vi "slm_control_MAIN.vi"() -> ()   [LabVIEW 2024]
uses:
  <vilib>/Python/Open Anaconda Python Session.vi
panel:
  in  "Send to SLM":bool=TRUE
  in  "stop_all":bool
  in  "Laser Wavelength":i32=635
  in  "SLM Cols":i32=800
  in  "SLM Rows":i32=600
  out "SLM Display":T1(plugin-control)
  in  "Tab Control":enum32{"Double Pass", "Single Pass"}(tab)
  in  "Linear Period Y":dbl
  in  "Linear Period X":dbl=4.0
  in  "Y Offset B":i32 min=-150 max=150 step=1
  in  "Y Offset A":i32 min=-150 max=150 step=1
  in  "X Offset A":i32 min=-150 max=150 step=1
  in  "B Display":bool=TRUE
  in  "A Display":bool=TRUE
  in  "Modulation Mode Double Pass":string(combo)
  in  "X Offset B":i32 min=-150 max=150 step=1
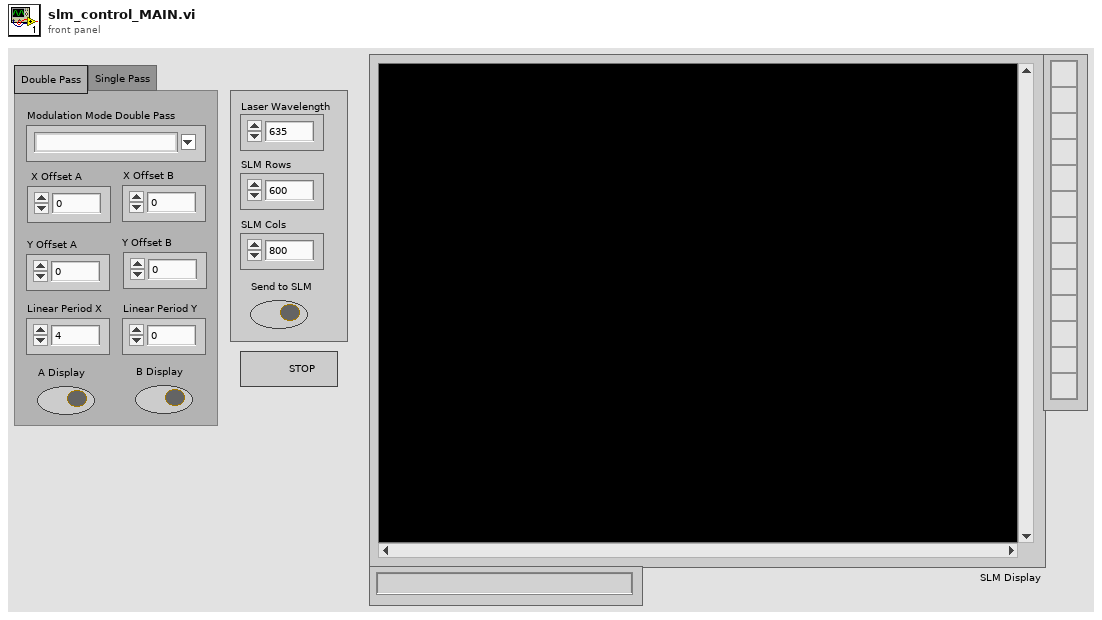
[diagram p1: front panel]
types:
  T1 = typedef "IMAQ Image.ctl" = refnum<image>
  T2 = enum16{"Init", "Idle", "Compute Modulation", "Stop All", "Shift Modulation"}
  T3 = enum16{"Init", "Idle", "Compute Modulation", "Stop All"}
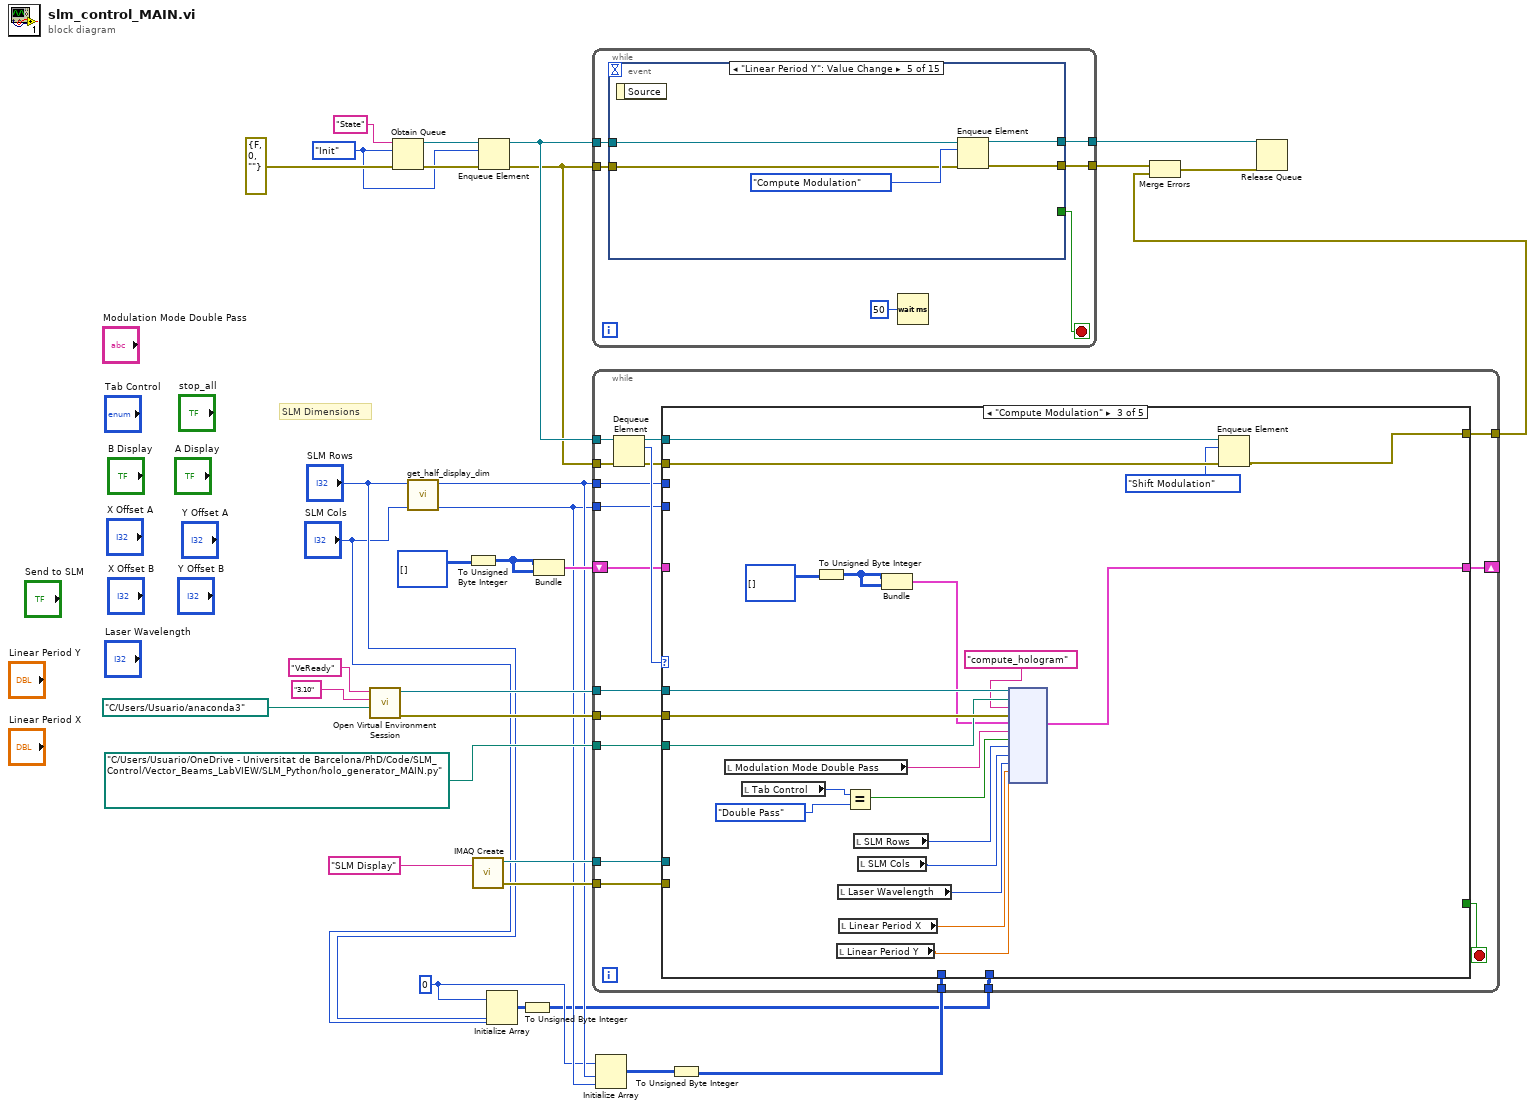
[diagram p0: block diagram]
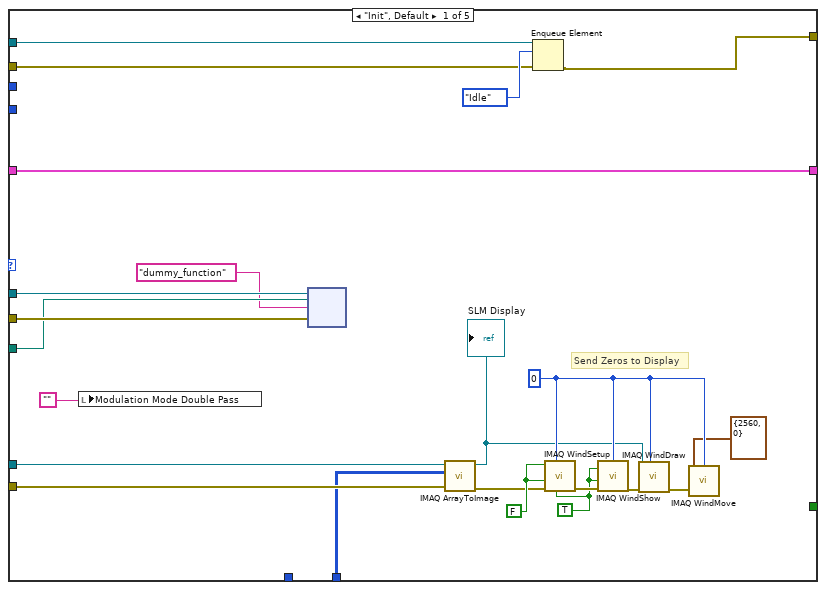
[diagram p2: hidden frame]
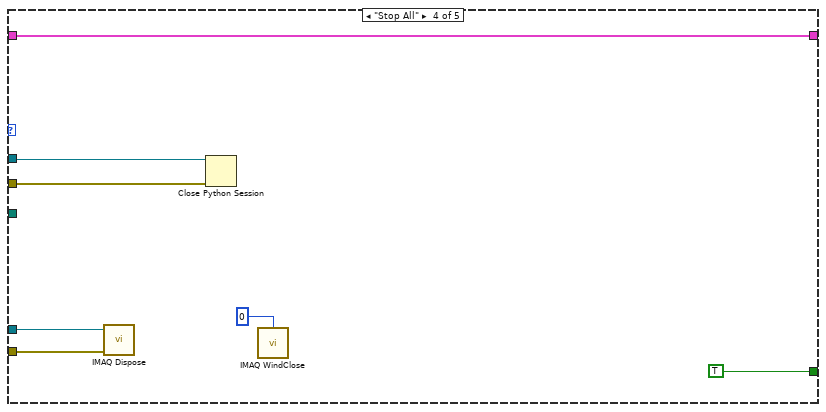
[diagram p4: hidden frame]
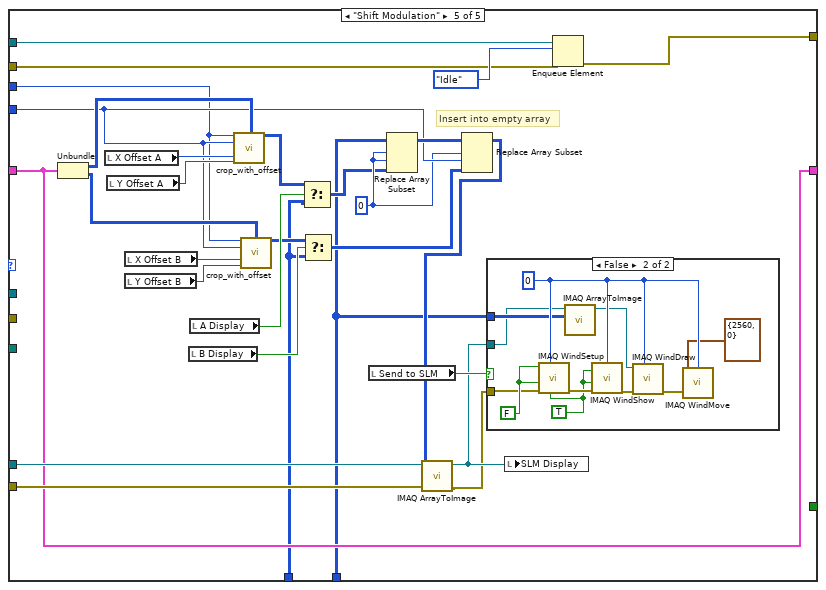
[diagram p5: hidden frame]
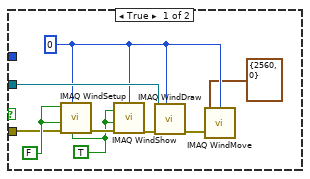
[diagram p6: hidden frame]
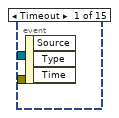
[diagram p7: hidden frame]
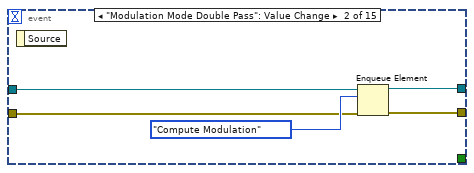
[diagram p8: hidden frame]
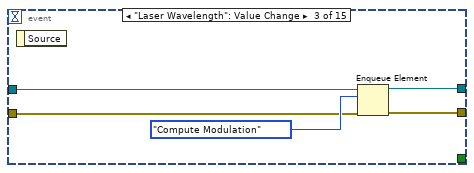
[diagram p9: hidden frame]
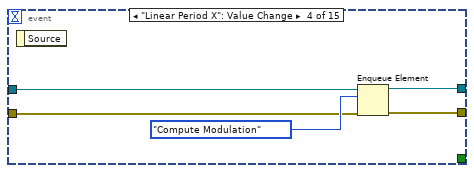
[diagram p10: hidden frame]
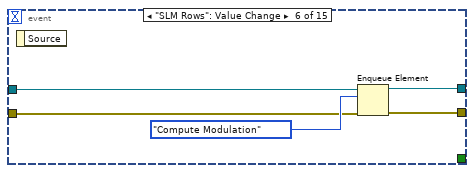
[diagram p11: hidden frame]
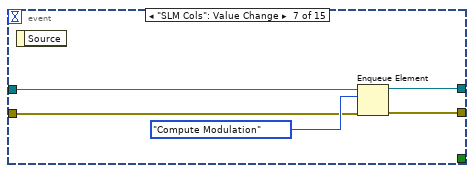
[diagram p12: hidden frame]
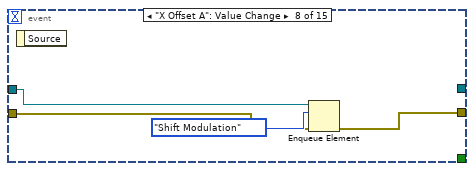
[diagram p13: hidden frame]
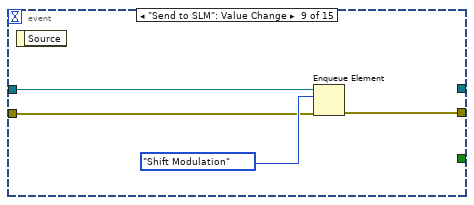
[diagram p14: hidden frame]
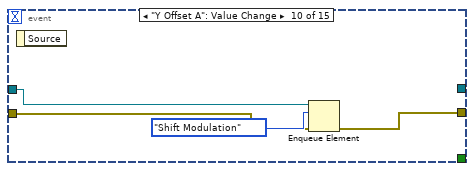
[diagram p15: hidden frame]
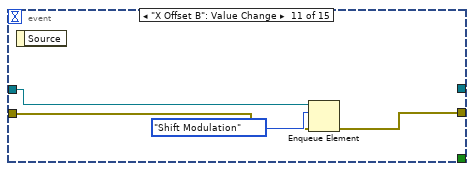
[diagram p16: hidden frame]
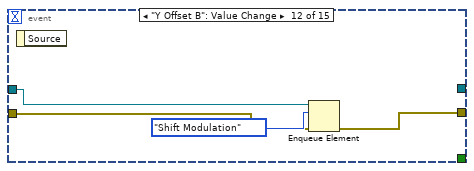
[diagram p17: hidden frame]
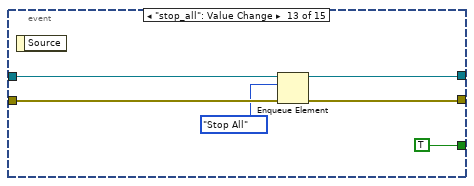
[diagram p18: hidden frame]
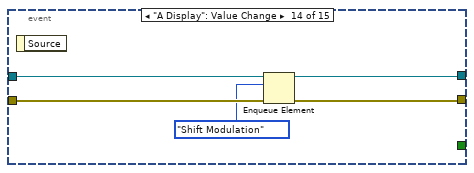
[diagram p19: hidden frame]
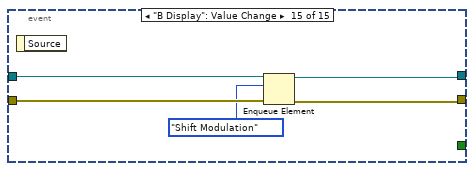
[diagram p20: hidden frame]
diagram:
  w5 = 0
  w9 = T2."Init"
  # "SLM Dimensions"
  n1 = call-poly <vilib>:"Open Virtual Environment Session.vi"("Anaconda path"=path "C:/Users/Usuario/anaconda3", "Python version"="3.10", "Env name"="VeReady") -> ("error out"=w23:errorcluster, "session out"=w24:refnum<k35>)  [unwired: 7 in]
  n2 = Obtain Queue(name (unnamed)="State", element data type=w9, error in (no error)=errorcluster {"status"=FALSE, "code"=0, "source"=""}) -> (queue out=w13:refnum<queue>, error out=w11:errorcluster)  [unwired: 2 in, 1 out]
  n3 = call "get_half_display_dim.vi"("Cols"="SLM Cols", "Rows"="SLM Rows") -> ("Semi Cols"=w6:i32, "Semi Rows"=w7:i32)  [unwired: 8 in]
  n4 = To Unsigned Byte Integer(number=i32[][] []) -> (unsigned 8bit integer=w16:u8[][])
  n5 = call "IMAQ Create"("Image Name"="SLM Display") -> ("New Image"=w19:T1, "error out"=w18:errorcluster)  [unwired: 4 in]
  n6 = Enqueue Element(queue=w13, element=w9, error in (no error)=w11) -> (queue out=w12:refnum<queue>, error out=w10:errorcluster)  [unwired: 1 in, 1 out]
  n7 = Initialize Array(w5, "SLM Rows", "SLM Cols") -> (w14:i32[][])
  n8 = To Unsigned Byte Integer(number=w14) -> (unsigned 8bit integer=w1:u8[][])
  n9 = Bundle(w16, w16) -> (w15:cluster{u8[][], u8[][]})  [unwired: 1 in]
  n10 = while {
    tunnel: w12 -> [w36]
    tunnel: [w35] -> w31
    tunnel: [w34] -> w29
    tunnel: w10 -> [w33]
    stop <- w37 stop-if-true
    n11 = event shown="[4] \"Linear Period Y\": Value Change" {
      selector: _ -> [_ _ _ _ _ _ _ _ _ _ _ _ _ _ _]
      dyn-events: _ -> [_ _ _ _ _ _ _ _ _ _ _ _ _ _ _]
      timeout: _ -> [_ _ _ _ _ _ _ _ _ _ _ _ _ _ _]
      tunnel: [_ _ _ _ _ _ _ _ _ _ _ _ TRUE _ _] -> w37
      tunnel: w36 -> [_ w43 w48 w53 w58 w63 w68 w71 w75 w79 w83 w87 w93 w99 w104]
      tunnel: [_ w42 w47 w52 w57 w62 w67 _ _ _ _ _ w90 w98 w103] -> w35
      tunnel: [_ w41 w46 w51 w56 w61 w66 w69 w73 w77 w81 w85 w91 w96 w101] -> w34
      tunnel: w33 -> [_ w39 w44 w49 w54 w59 w64 w70 w74 w78 w82 w86 w92 w97 w102]
      event Timeout {
        n12 = event-data() -> ()  [unwired: 1 in, 3 out]
      }
      event "Modulation Mode Double Pass": Value Change {
        n13 = event-data() -> ()  [unwired: 1 in, 1 out]
        n14 = Enqueue Element(queue=w43, element=enum16{"Init", "Idle", "Compute Modulation"}."Compute Modulation", error in (no error)=w39) -> (queue out=w42:refnum<queue>, error out=w41:errorcluster)  [unwired: 1 in, 1 out]
      }
      event "Laser Wavelength": Value Change {
        n15 = event-data() -> ()  [unwired: 1 in, 1 out]
        n16 = Enqueue Element(queue=w48, element=enum16{"Init", "Idle", "Compute Modulation"}."Compute Modulation", error in (no error)=w44) -> (queue out=w47:refnum<queue>, error out=w46:errorcluster)  [unwired: 1 in, 1 out]
      }
      event "Linear Period X": Value Change {
        n17 = event-data() -> ()  [unwired: 1 in, 1 out]
        n18 = Enqueue Element(queue=w53, element=enum16{"Init", "Idle", "Compute Modulation"}."Compute Modulation", error in (no error)=w49) -> (queue out=w52:refnum<queue>, error out=w51:errorcluster)  [unwired: 1 in, 1 out]
      }
      event "Linear Period Y": Value Change {
        n19 = event-data() -> ()  [unwired: 1 in, 1 out]
        n20 = Enqueue Element(queue=w58, element=enum16{"Init", "Idle", "Compute Modulation"}."Compute Modulation", error in (no error)=w54) -> (queue out=w57:refnum<queue>, error out=w56:errorcluster)  [unwired: 1 in, 1 out]
      }
      event "SLM Rows": Value Change {
        n21 = event-data() -> ()  [unwired: 1 in, 1 out]
        n22 = Enqueue Element(queue=w63, element=enum16{"Init", "Idle", "Compute Modulation"}."Compute Modulation", error in (no error)=w59) -> (queue out=w62:refnum<queue>, error out=w61:errorcluster)  [unwired: 1 in, 1 out]
      }
      event "SLM Cols": Value Change {
        n23 = event-data() -> ()  [unwired: 1 in, 1 out]
        n24 = Enqueue Element(queue=w68, element=enum16{"Init", "Idle", "Compute Modulation"}."Compute Modulation", error in (no error)=w64) -> (queue out=w67:refnum<queue>, error out=w66:errorcluster)  [unwired: 1 in, 1 out]
      }
      event "X Offset A": Value Change {
        n25 = event-data() -> ()  [unwired: 1 in, 1 out]
        n26 = Enqueue Element(queue=w71, element=T2."Shift Modulation", error in (no error)=w70) -> (error out=w69:errorcluster)  [unwired: 1 in, 2 out]
      }
      event "Send to SLM": Value Change {
        n27 = event-data() -> ()  [unwired: 1 in, 1 out]
        n28 = Enqueue Element(queue=w75, element=T2."Shift Modulation", error in (no error)=w74) -> (error out=w73:errorcluster)  [unwired: 1 in, 2 out]
      }
      event "Y Offset A": Value Change {
        n29 = event-data() -> ()  [unwired: 1 in, 1 out]
        n30 = Enqueue Element(queue=w79, element=T2."Shift Modulation", error in (no error)=w78) -> (error out=w77:errorcluster)  [unwired: 1 in, 2 out]
      }
      event "X Offset B": Value Change {
        n31 = event-data() -> ()  [unwired: 1 in, 1 out]
        n32 = Enqueue Element(queue=w83, element=T2."Shift Modulation", error in (no error)=w82) -> (error out=w81:errorcluster)  [unwired: 1 in, 2 out]
      }
      event "Y Offset B": Value Change {
        n33 = event-data() -> ()  [unwired: 1 in, 1 out]
        n34 = Enqueue Element(queue=w87, element=T2."Shift Modulation", error in (no error)=w86) -> (error out=w85:errorcluster)  [unwired: 1 in, 2 out]
      }
      event "stop_all": Value Change {
        n35 = event-data() -> ()  [unwired: 1 in, 1 out]
        n36 = Enqueue Element(queue=w93, element=T3."Stop All", error in (no error)=w92) -> (queue out=w90:refnum<queue>, error out=w91:errorcluster)  [unwired: 1 in, 1 out]
      }
      event "A Display": Value Change {
        n37 = event-data() -> ()  [unwired: 1 in, 1 out]
        n38 = Enqueue Element(queue=w99, element=T2."Shift Modulation", error in (no error)=w97) -> (queue out=w98:refnum<queue>, error out=w96:errorcluster)  [unwired: 1 in, 1 out]
      }
      event "B Display": Value Change {
        n39 = event-data() -> ()  [unwired: 1 in, 1 out]
        n40 = Enqueue Element(queue=w104, element=T2."Shift Modulation", error in (no error)=w102) -> (queue out=w103:refnum<queue>, error out=w101:errorcluster)  [unwired: 1 in, 1 out]
      }
    }
    n41 = Wait (ms)(milliseconds to wait=u32 50) -> ()  [unwired: 1 out]
  }
  n42 = Initialize Array(w5, w7, w6) -> (w8:i32[][])
  n43 = To Unsigned Byte Integer(number=w8) -> (unsigned 8bit integer=w4:u8[][])
  n44 = while {
    tunnel: w12 -> [w122]
    tunnel: w10 -> [w121]
    tunnel: [w119] -> w30
    tunnel: w24 -> [w116]
    tunnel: w23 -> [w115]
    tunnel: path "C:/Users/Usuario/OneDrive - Universitat de Barcelona/PhD/Code/SLM_Control/Vector_Beams_LabVIEW/SLM_Python/holo_generator_MAIN.py" ("module path") -> [w114]
    tunnel: w19 -> [w112]
    tunnel: w18 -> [w111]
    shift-right: [w110] -> _
    shift-left: w15 -> [w109]
    tunnel: w7 -> [w108]
    tunnel: w1 -> [w107]
    tunnel: w6 -> [w106]
    tunnel: w4 -> [w105]
    stop <- w117 stop-if-true
    n45 = Dequeue Element(queue=w122, error in (no error)=w121) -> (queue out=w113:refnum<queue>, element=w120:T2, error out=w118:errorcluster)  [unwired: 1 in, 1 out]
    n46 = case shown="\"Compute Modulation\"" w120 {
      tunnel: [w141 _ w159 _ w196] -> w119
      tunnel: w118 -> [w143 _ w161 _ w197]
      tunnel: [_ _ _ TRUE _] -> w117
      tunnel: w116 -> [w139 _ w166 w172 _]
      tunnel: w115 -> [w138 _ w165 w171 _]
      tunnel: w114 -> [w137 _ w164 _ _]
      tunnel: w113 -> [w142 _ w160 _ w198]
      tunnel: w112 -> [w135 _ _ w170 w202]
      tunnel: w111 -> [w134 _ _ w169 w201]
      tunnel: [w140 w145 w151 w168 w195] -> w110
      tunnel: w109 -> [w140 w145 _ w168 w195]
      tunnel: w108 -> [_ _ _ _ w186]
      tunnel: w107 -> [w133 _ _ _ w174]
      tunnel: w106 -> [_ _ _ _ w190]
      tunnel: w105 -> [_ _ _ _ w180]
      frame "Init", Default {
        w131 = TRUE ("Window has title bar? (Yes)")
        w130 = FALSE ("Window has title bar? (Yes)")
        w129 = 0 ("Window Number (0...15)")
        # "Send Zeros to Display"
        n47 = local write "Modulation Mode Double Pass"("") -> ()
        n48 = node(w139, w137, "dummy_function" ("function name"), w138) -> ()  [unwired: 2 in, 4 out]
        n49 = call "IMAQ ArrayToImage"("error in (no error)"=w134, "Image Pixels (U8)"=w133, "Image"=w135) -> ("error out"=w125:errorcluster, "Image Out"=w124:T1)  [unwired: 7 in]
        "SLM Display" <- w124
        n50 = Enqueue Element(queue=w142, element=T3."Idle", error in (no error)=w143) -> (error out=w141:errorcluster)  [unwired: 1 in, 2 out]
        n51 = call "IMAQ WindSetup"("Window is floating? (No)"=w131, "Window Number (0...15)"=w129, "error in (no error)"=w125, "Window has title bar? (Yes)"=w130, "Window can grow? (Yes)"=w130) -> ("error out"=w132:errorcluster)  [unwired: 6 in]
        n52 = call "IMAQ WindShow"("error in (no error)"=w132, "Bring To Front? (N)"=w131, "Hide/Show (Show)"=w131, "Window Number (0...15)"=w129) -> ("error out"=w126:errorcluster)  [unwired: 2 in, 2 out]
        n53 = call "IMAQ WindDraw"("Window Number (0...15)"=w129, "error in (no error)"=w126, "Image"=w124) -> ("error out"=w127:errorcluster)  [unwired: 7 in, 1 out]
        n54 = call "IMAQ WindMove"("Window Number (0...15)"=w129, "Coordinates (screen)"=cluster{"X Position":i32, "Y Position":i32} {"X Position"=2560, "Y Position"=0}, "error in (no error)"=w127) -> ()  [unwired: 2 in, 2 out]
      }
      frame "Idle" {
      }
      frame "Compute Modulation" {
        n55 = local read "Modulation Mode Double Pass"() -> (w163:string)
        n56 = local read "Tab Control"() -> (w158:enum32{"Double Pass", "Single Pass"})
        n57 = To Unsigned Byte Integer(number=i32[][] []) -> (unsigned 8bit integer=w154:u8[][])
        n58 = local read "Linear Period Y"() -> (w146:dbl)
        n59 = local read "Laser Wavelength"() -> (w148:i32)
        n60 = local read "Linear Period X"() -> (w147:dbl)
        n61 = Equal?(x=w158, y=enum32{"Double Pass", "Single Pass"}."Double Pass") -> (x = y?=w156:bool)
        n62 = local read "SLM Rows"() -> (w150:i32)
        n63 = local read "SLM Cols"() -> (w149:i32)
        n64 = Bundle(w154, w154) -> (w153:cluster{u8[][], u8[][]})  [unwired: 1 in]
        n65 = node(w166, w164, "compute_hologram" ("function name"), w165, w153, w163, w156, w150, w149, w148, w147, w146) -> (w151:cluster{u8[][], u8[][]})  [unwired: 7 in, 4 out]
        n66 = Enqueue Element(queue=w160, element=T2."Shift Modulation", error in (no error)=w161) -> (error out=w159:errorcluster)  [unwired: 1 in, 2 out]
      }
      frame "Stop All" {
        n67 = call "IMAQ Dispose"("Image"=w170, "error in (no error)"=w169) -> ()  [unwired: 1 in, 4 out]
        n68 = Close Python Session(session in=w172, error in=w171) -> ()  [unwired: 1 out]
        n69 = call "IMAQ WindClose"("Window Number (0...15)"=0) -> ()  [unwired: 5 in, 1 out]
      }
      frame "Shift Modulation" {
        w187 = 0 ("index (row)")
        # "Insert into empty array"
        n70 = Unbundle(w195) -> (w194:u8[][], w191:u8[][])
        n71 = local read "X Offset A"() -> (w192:i32)
        n72 = local read "Y Offset A"() -> (w193:i32)
        n73 = local read "X Offset B"() -> (w189:i32)
        n74 = local read "Y Offset B"() -> (w188:i32)
        n75 = local read "B Display"() -> (w182:bool)
        n76 = local read "A Display"() -> (w185:bool)
        n77 = call "crop_with_offset.vi"("Out Rows"=w186, "Array"=w194, "Out Cols"=w190, "Offset X"=w192, "Offset Y"=w193) -> ("subarray"=w183:i32[][])  [unwired: 10 in]
        n78 = call "crop_with_offset.vi"("Out Rows"=w186, "Array"=w191, "Out Cols"=w190, "Offset X"=w189, "Offset Y"=w188) -> ("subarray"=w181:i32[][])  [unwired: 10 in]
        n79 = Select(t=w183, s=w185, f=w180) -> (s? t:f=w184:i32[][])
        n80 = Select(t=w181, s=w182, f=w180) -> (s? t:f=w179:i32[][])
        n81 = local read "Send to SLM"() -> (w178:bool)
        n82 = Replace Array Subset(array=w174, new element=w184, index (row)=w187, index (col)=w187) -> (w200:u8[][])
        n83 = Replace Array Subset(array=w200, new element=w179, index (row)=w187, index (col)=w190) -> (w175:u8[][])
        n84 = call "IMAQ ArrayToImage"("error in (no error)"=w201, "Image Pixels (U8)"=w175, "Image"=w202) -> ("error out"=w176:errorcluster, "Image Out"=w177:T1)  [unwired: 7 in]
        n85 = case shown="False" w178 {
          tunnel: w177 -> [w210 w212]
          tunnel: w176 -> [w205 w217]
          tunnel: w174 -> [_ w214]
          frame True {
            w209 = TRUE ("Window has title bar? (Yes)")
            w208 = FALSE ("Window has title bar? (Yes)")
            w207 = 0 ("Window Number (0...15)")
            n86 = call "IMAQ WindSetup"("Window is floating? (No)"=w209, "Window Number (0...15)"=w207, "error in (no error)"=w205, "Window has title bar? (Yes)"=w208, "Window can grow? (Yes)"=w208) -> ("error out"=w211:errorcluster)  [unwired: 6 in]
            n87 = call "IMAQ WindShow"("error in (no error)"=w211, "Bring To Front? (N)"=w209, "Hide/Show (Show)"=w209, "Window Number (0...15)"=w207) -> ("error out"=w203:errorcluster)  [unwired: 2 in, 2 out]
            n88 = call "IMAQ WindDraw"("Window Number (0...15)"=w207, "error in (no error)"=w203, "Image"=w210) -> ("error out"=w204:errorcluster)  [unwired: 7 in, 1 out]
            n89 = call "IMAQ WindMove"("Window Number (0...15)"=w207, "Coordinates (screen)"=cluster{"X Position":i32, "Y Position":i32} {"X Position"=2560, "Y Position"=0}, "error in (no error)"=w204) -> ()  [unwired: 2 in, 2 out]
          }
          frame False {
            w221 = TRUE ("Window has title bar? (Yes)")
            w220 = FALSE ("Window has title bar? (Yes)")
            w219 = 0 ("Window Number (0...15)")
            n90 = call "IMAQ WindSetup"("Window is floating? (No)"=w221, "Window Number (0...15)"=w219, "error in (no error)"=w217, "Window has title bar? (Yes)"=w220, "Window can grow? (Yes)"=w220) -> ("error out"=w222:errorcluster)  [unwired: 6 in]
            n91 = call "IMAQ ArrayToImage"("Image Pixels (U8)"=w214, "Image"=w212) -> ("Image Out"=w213:T1)  [unwired: 8 in, 1 out]
            n92 = call "IMAQ WindShow"("error in (no error)"=w222, "Bring To Front? (N)"=w221, "Hide/Show (Show)"=w221, "Window Number (0...15)"=w219) -> ("error out"=w215:errorcluster)  [unwired: 2 in, 2 out]
            n93 = call "IMAQ WindDraw"("Window Number (0...15)"=w219, "error in (no error)"=w215, "Image"=w213) -> ("error out"=w216:errorcluster)  [unwired: 7 in, 1 out]
            n94 = call "IMAQ WindMove"("Window Number (0...15)"=w219, "Coordinates (screen)"=cluster{"X Position":i32, "Y Position":i32} {"X Position"=2560, "Y Position"=0}, "error in (no error)"=w216) -> ()  [unwired: 2 in, 2 out]
          }
        }
        n95 = local write "SLM Display"(w177) -> ()
        n96 = Enqueue Element(queue=w198, element=T2."Idle", error in (no error)=w197) -> (error out=w196:errorcluster)  [unwired: 1 in, 2 out]
      }
    }
  }
  n97 = Merge Errors(w29, w30) -> (w28:errorcluster)
  n98 = Release Queue(queue=w31, error in (no error)=w28) -> ()  [unwired: 1 in, 3 out]
